vi "State from Values.vi"() -> ()   [LabVIEW 2017]
panel:
  in  "Desired State":i32
  in  "Elbow Brake":bool=TRUE
  in  "Shoulder Brake":bool=TRUE
  in  "Current Shoulder\nAngle (Rad)":dbl
  in  "Current Shoulder\nAngle (Rad)":dbl
  out "State":i32
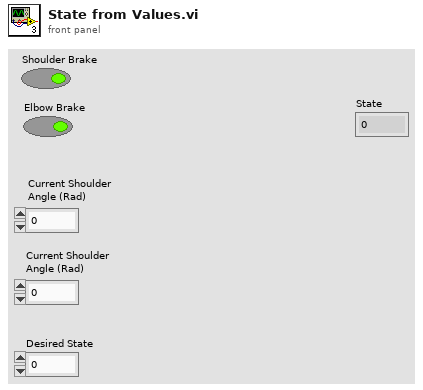
[diagram p1: front panel]
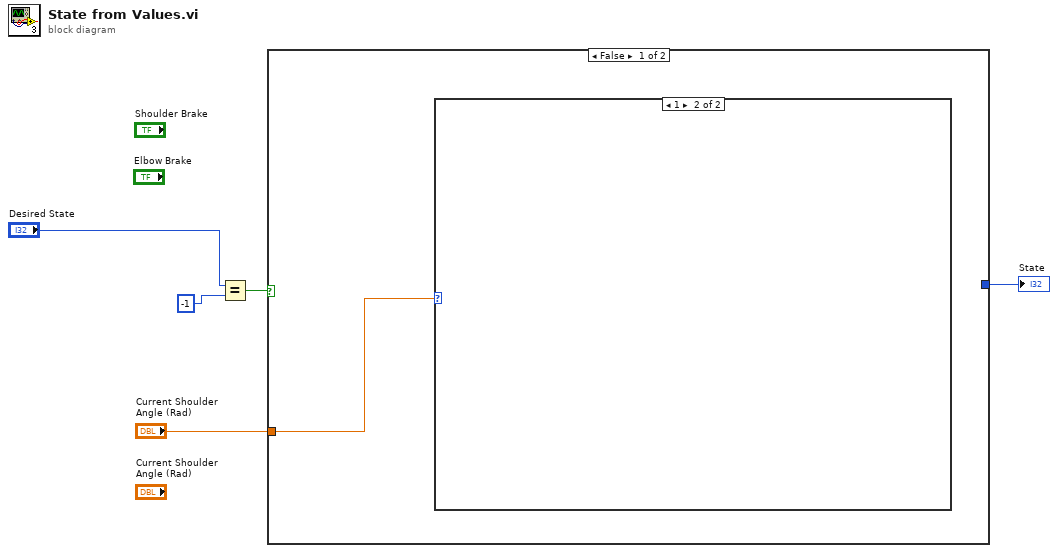
[diagram p0: block diagram]
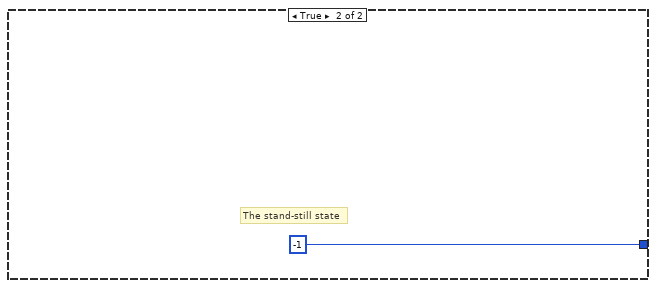
[diagram p3: hidden frame]
diagram:
  n1 = Equal?(x="Desired State", y=-1) -> (x = y?=w5:bool)
  n2 = case shown="False" w5 {
    tunnel: [_ -1] -> w2
    tunnel: "Current Shoulder\nAngle (Rad)" -> [w6 _]
    frame False {
      n3 = case shown="1" w6 {
        frame 0, Default {
        }
        frame 1 {
        }
      }
    }
    frame True {
      # "The stand-still state"
    }
  }
  "State" <- w2
